vi "drive dual picomotor zigzag (SubVI).vi"(10 "Picomotor Index":i32, 11 "Picomotor Cluster":T2) -> (3 "Picomotor Instr Out":T1)   [LabVIEW 2014]
uses:
  C:/Program Files/National Instruments/LabVIEW 2014/instr.lib/Model 8742/CmdLib.dll
  Program Files/National Instruments/LabVIEW 2014/instr.lib/Model 8742/CmdLib.dll
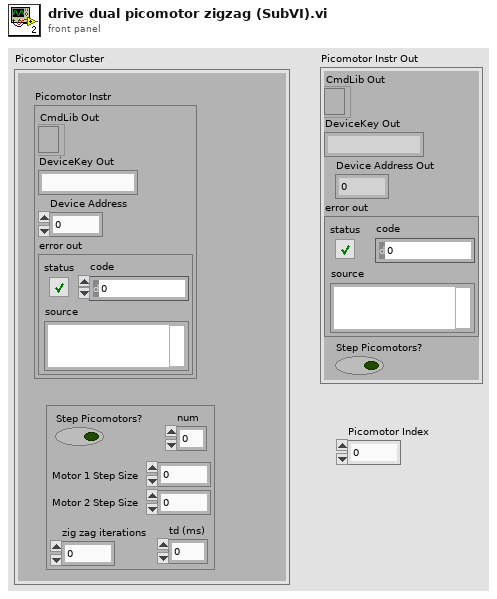
[diagram p1: front panel]
types:
  T1 = cluster{"CmdLib Out":refnum<k24>, "DeviceKey Out":string, "Device Address Out":i32, "error out":errorcluster, "Step Picomotors?":bool}
  T2 = cluster{"Picomotor Instr":cluster{"CmdLib Out":refnum<k24>, "DeviceKey Out":string, "Device Address":i32, "error out":errorcluster}, "Picomotor Stepping":cluster{"Motor 1 Step Size":i32, "zig zag iterations":i32, "Motor 2 Step Size":i32, "Step Picomotors?":bool, "td (ms)":dbl, "num":i32}}
  T3 = cluster{"CmdLib Out":refnum<k24>, "DeviceKey Out":string, "Device Address":i32, "error out":errorcluster}
  T4 = cluster{"Motor 1 Step Size":i32, "zig zag iterations":i32, "Motor 2 Step Size":i32, "Step Picomotors?":bool, "td (ms)":dbl, "num":i32}
  T5 = cluster{"CmdLib Out":refnum<k24>, "DeviceKey Out":string, "Device Address":i32, "error out":errorcluster, "Step Picomotors?":bool}
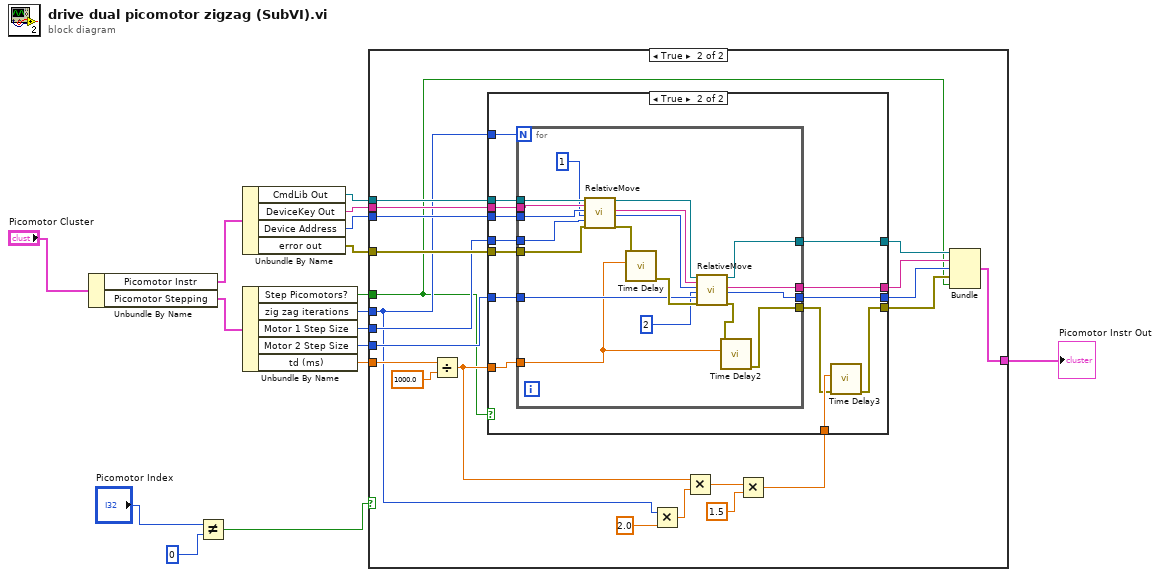
[diagram p0: block diagram]
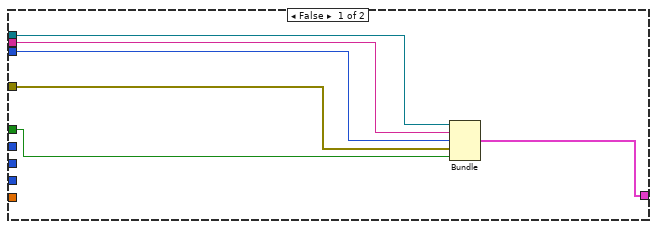
[diagram p2: hidden frame]
diagram:
  n1 = Unbundle By Name("Picomotor Cluster") -> ("Picomotor Instr"=w15:T3, "Picomotor Stepping"=w10:T4)
  n2 = Not Equal?(x="Picomotor Index", y=0) -> (x != y?=w3:bool)
  n3 = Unbundle By Name(w15) -> ("CmdLib Out"=w14:refnum<k24>, "DeviceKey Out"=w13:string, "Device Address"=w12:i32, "error out"=w11:errorcluster)
  n4 = Unbundle By Name(w10) -> ("Step Picomotors?"=w4:bool, "zig zag iterations"=w5:i32, "Motor 1 Step Size"=w9:i32, "Motor 2 Step Size"=w8:i32, "td (ms)"=w6:dbl)
  n5 = case shown="True" w3 {
    tunnel: w14 -> [w21 w43]
    tunnel: w13 -> [w20 w42]
    tunnel: w12 -> [w19 w41]
    tunnel: w11 -> [w18 w40]
    tunnel: w9 -> [_ w39]
    tunnel: w8 -> [_ w38]
    tunnel: [w17 w34] -> w7
    tunnel: w6 -> [_ w32]
    tunnel: w5 -> [_ w29]
    tunnel: w4 -> [w22 w23]
    frame False {
      n6 = Bundle("CmdLib Out"=w21, "DeviceKey Out"=w20, "Device Address"=w19, "error out"=w18, "Step Picomotors?"=w22) -> (w17:T5)  [unwired: 1 in]
    }
    frame True {
      n7 = Divide(x=w32, y=1000.0) -> (x/y=w28:dbl)
      n8 = Multiply(x=w29, y=2.0) -> (x*y=w30:dbl)
      n9 = Multiply(x=w28, y=w30) -> (x*y=w27:dbl)
      n10 = Multiply(x=w27, y=1.5) -> (x*y=w25:dbl)
      n11 = case shown="True" w23 {
        tunnel: w43 -> [w47 w61]
        tunnel: w42 -> [w46 w60]
        tunnel: w41 -> [w45 w59]
        tunnel: w40 -> [w44 w58]
        tunnel: [w47 w57] -> w37
        tunnel: [w46 w56] -> w36
        tunnel: [w45 w55] -> w35
        tunnel: w29 -> [_ w54]
        tunnel: w39 -> [_ w53]
        tunnel: w38 -> [_ w52]
        tunnel: w28 -> [_ w51]
        tunnel: w25 -> [_ w50]
        tunnel: [w44 w48] -> w24
        frame False {
        }
        frame True {
          n12 = for {
            N: w54 -> [_]
            tunnel: w61 -> [w75]
            tunnel: w60 -> [w74]
            tunnel: w59 -> [w73]
            tunnel: w58 -> [w72]
            tunnel: [w71] -> w57
            tunnel: [w70] -> w56
            tunnel: [w69] -> w55
            tunnel: [w67] -> w49
            tunnel: w53 -> [w65]
            tunnel: w52 -> [w64]
            tunnel: w51 -> [w62]
            n13 = call <instrlib>:"RelativeMove.vi"("CmdLib In"=w75, "DeviceKey In"=w74, "Device Address In"=w73, "Motor"=1, "Relative Steps"=w65, "error in (no error)"=w72) -> ("CmdLib Out"=w80:refnum<k24>, "DeviceKey Out"=w79:string, "Device Address Out"=w78:i32, "error out"=w77:errorcluster)  [unwired: 10 in]
            n14 = call "Time Delay"("error in (no error)"=w77, "Delay Time (s)"=w62) -> ("error out"=w76:errorcluster)  [unwired: 9 in]
            n15 = call <instrlib>:"RelativeMove.vi"("CmdLib In"=w80, "DeviceKey In"=w79, "Device Address In"=w78, "Motor"=2, "Relative Steps"=w64, "error in (no error)"=w76) -> ("CmdLib Out"=w71:refnum<k24>, "DeviceKey Out"=w70:string, "Device Address Out"=w69:i32, "error out"=w68:errorcluster)  [unwired: 10 in]
            n16 = call "Time Delay2"("error in (no error)"=w68, "Delay Time (s)"=w62) -> ("error out"=w67:errorcluster)  [unwired: 9 in]
          }
          n17 = call "Time Delay3"("error in (no error)"=w49, "Delay Time (s)"=w50) -> ("error out"=w48:errorcluster)  [unwired: 9 in]
        }
      }
      n18 = Bundle("CmdLib Out"=w37, "DeviceKey Out"=w36, "Device Address Out"=w35, "error out"=w24, "Step Picomotors?"=w23) -> (w34:T1)  [unwired: 1 in]
    }
  }
  "Picomotor Instr Out" <- w7
